vi "Set motor start time.vi"(7 "t0":timestamp, 10 "stimphases":T1, 11 "motor in":waveform(dbl)) -> (2 "stimphases out":T1, 3 "motor out":waveform(dbl))   [LabVIEW 2013]
uses:
  Stim phases.ctl
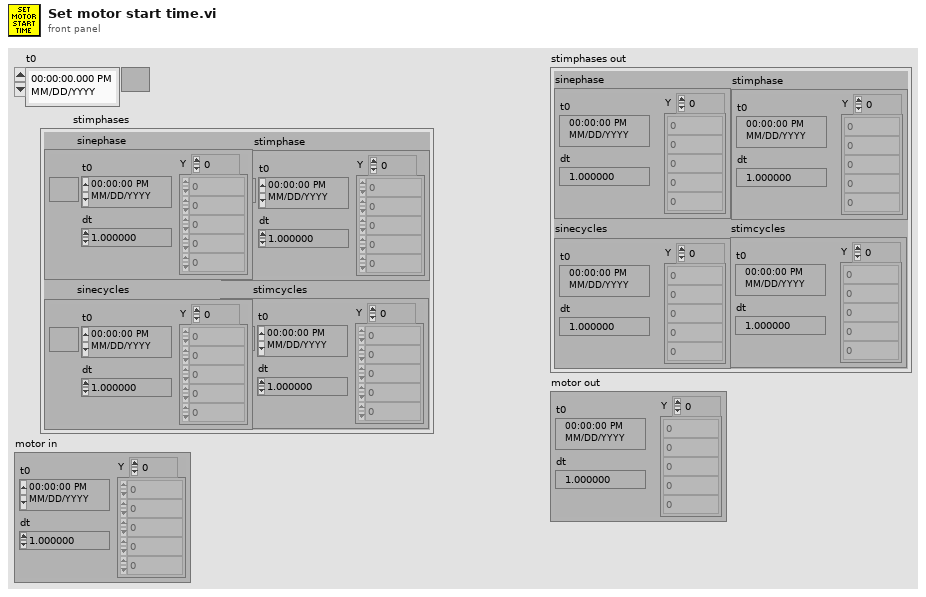
[diagram p1: front panel]
types:
  T1 = typedef "Stim phases.ctl" = cluster{"sinephase":waveform(dbl), "sinecycles":waveform(dbl), "stimphase":waveform(dbl), "stimcycles":waveform(dbl)}
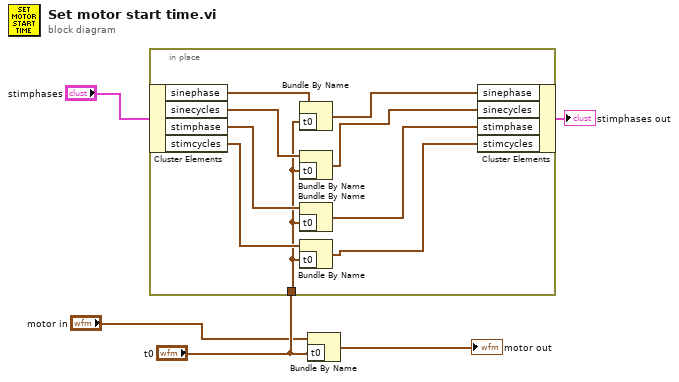
[diagram p0: block diagram]
diagram:
  n1 = in-place {
    in-place-border: "t0" -> [w10]
    n2 = in-place-cluster #1("stimphases") -> ("sinephase"=w14:waveform(dbl), "sinecycles"=w13:waveform(dbl), "stimphase"=w12:waveform(dbl), "stimcycles"=w11:waveform(dbl))
    n3 = Bundle By Name(cluster=w14, "t0"=w10) -> (w9:waveform(dbl))
    n4 = Bundle By Name(cluster=w13, "t0"=w10) -> (w8:waveform(dbl))
    n5 = Bundle By Name(cluster=w12, "t0"=w10) -> (w7:waveform(dbl))
    n6 = Bundle By Name(cluster=w11, "t0"=w10) -> (w6:waveform(dbl))
    n7 = in-place-cluster #1("sinephase"=w9, "sinecycles"=w8, "stimphase"=w7, "stimcycles"=w6) -> (→"stimphases out":T1)
  }
  n8 = Bundle By Name(cluster="motor in", "t0"="t0") -> (→"motor out":waveform(dbl))
